vi "Fold.vi"() -> ()   [LabVIEW 2020, in "Examples.lvlib"]
doc: "Example that showcases how to use Fold with strings by folding an array of strings to strings on new lines in a single string."
uses:
  Examples.lvlib
  6b1d3035-d609-4a69-ab56-06123d6e7127.vi
panel:
  out "Final State":string
  in  "Array":string[](array[string])=["[Person]", "first-name = Jim", "last-name = Bob", "age = 31"]
  # "1) Take note of the existing strings in the Array control. Add new ones if you would like. These are meant to mimic lines in an INI file.\n2) Run the VI.\n3) Note that the Final State has taken the lines and put them on a new line of a text string, ready to be written to an INI file.\n4) View the block diagram."
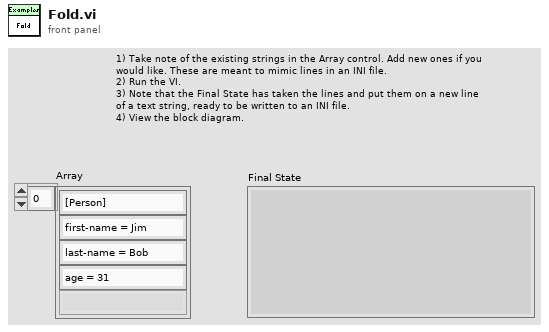
[diagram p1: front panel]
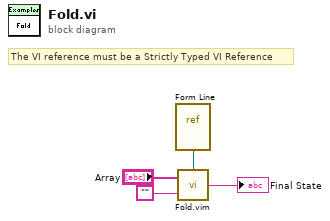
[diagram p0: block diagram]
diagram:
  # "The VI reference must be a Strictly Typed VI Reference"
  n1 = vi-ref "Form Line.vi"() -> (w4:refnum<vi>)
  n2 = call "Fold.vim"("Processor"=w4, "Initial State"="", "Array"="Array") -> ("Final State"=→"Final State":string)
